vi "Get Waveform Data.vi"(8 "error in (no error)":errorcluster, 10 "Waveform to Retrieve":string, 11 "QPA Measurement in":refnum<class "QPA Measurement.lvclass">) -> (0 "error out":errorcluster, 2 "RF Waveform":T1, 3 "QPA Measurement out":refnum<class "QPA Measurement.lvclass">)   [LabVIEW 2014, in "QPA Measurement.lvlib" / "QPA Measurement.lvclass"]
uses:
  QPA Measurement.lvclass
  Controls/RF Waveform.ctl
  QPA Measurement.lvclass/QPA Measurement.ctl
  Read RF Waveform Database.vi
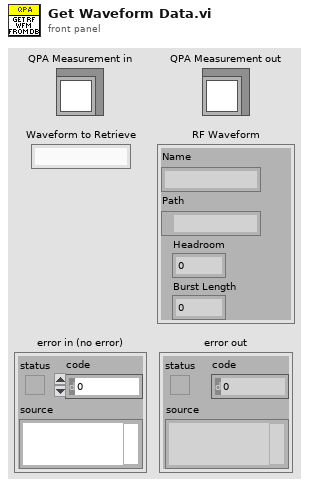
[diagram p1: front panel]
types:
  T1 = typedef "QPA Measurement.lvlib/QPA Measurement.lvclass/RF Waveform.ctl" = cluster{"Name":string, "Path":path, "Headroom":dbl, "Burst Length":dbl}
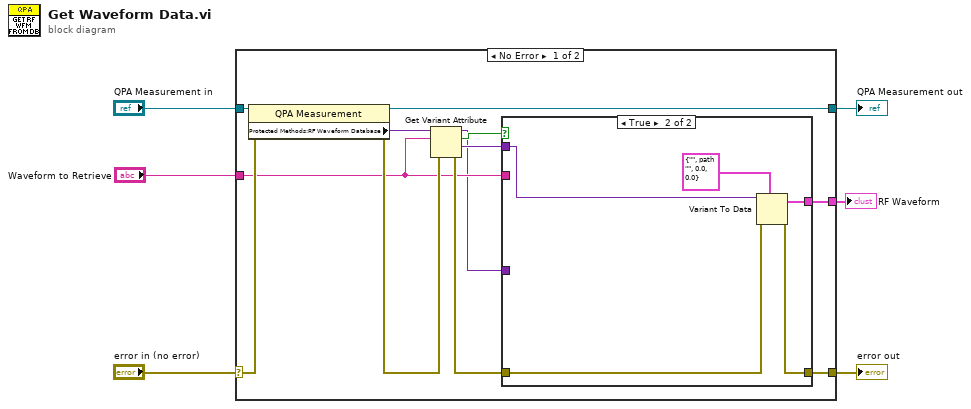
[diagram p0: block diagram]
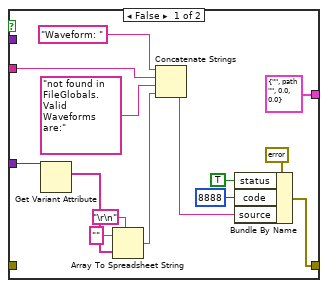
[diagram p2: hidden frame]
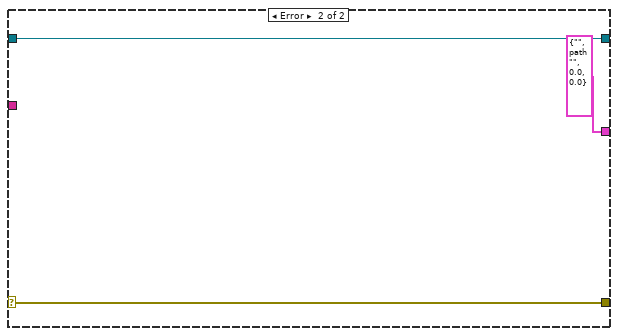
[diagram p3: hidden frame]
diagram:
  n1 = case shown="No Error" "error in (no error)" {
    selector: "error in (no error)" -> [w18 w40]
    tunnel: [w12 w40] -> w5
    tunnel: [w16 w39] -> w3
    tunnel: "QPA Measurement in" -> [w17 w39]
    tunnel: [w10 T1 {"Name"="", "Path"=path "", "Headroom"=0.0, "Burst Length"=0.0} ("RF Waveform")] -> w2
    tunnel: "Waveform to Retrieve" -> [w8 _]
    frame No Error {
      n2 = property class="QPA Measurement"(reference=w17, error in=w18) -> (reference out=w16:refnum<class "QPA Measurement.lvclass">, error out=w13:errorcluster, "Protected Methods:RF Waveform Database"=w15:variant)
      n3 = Get Variant Attribute(Variant=w15, name=w8, error in=w13) -> (duplicate Variant=w7:variant, found=w9:bool, value=w11:variant, error out=w14:errorcluster)  [unwired: 1 in]
      n4 = case shown="True" w9 {
        tunnel: w14 -> [_ w37]
        tunnel: [w31 w36] -> w12
        tunnel: w11 -> [_ w35]
        tunnel: [T1 {"Name"="", "Path"=path "", "Headroom"=0.0, "Burst Length"=0.0} ("RF Waveform") w34] -> w10
        tunnel: w8 -> [w26 _]
        tunnel: w7 -> [w24 _]
        frame False {
          n5 = Get Variant Attribute(Variant=w24) -> (names=w23:string[])  [unwired: 3 in, 3 out]
          n6 = Array To Spreadsheet String(delimiter (Tab)="\r\n", array=w23, 3:"" ("format string")) -> (spreadsheet string=w21:string)
          n7 = Concatenate Strings("Waveform: " ("source"), w26, "not found in FileGlobals.  Valid Waveforms are:" ("string"), w21) -> (w20:string)
          n8 = Bundle By Name(cluster=errorcluster {"status"=FALSE, "code"=0, "source"=""} ("error out"), "status"=TRUE, "code"=8888, "source"=w20) -> (w31:errorcluster)
        }
        frame True {
          n9 = Variant To Data(error in=w37, type=T1 {"Name"="", "Path"=path "", "Headroom"=0.0, "Burst Length"=0.0} ("RF Waveform"), Variant=w35) -> (data=w34:T1, error out=w36:errorcluster)
        }
      }
    }
    frame Error {
    }
  }
  "error out" <- w5
  "QPA Measurement out" <- w3
  "RF Waveform" <- w2
